vi "Get TDMS File Groups and Channels.vi"(8 "error in":errorcluster, 11 "TDMS ref in":refnum<k34>) -> (0 "error out":errorcluster, 2 "file contents":cluster{string, string[]}[](array[cluster]), 3 "TDMS ref out":refnum<k34>)   [LabVIEW 2020, in "TdmsFileViewer.lvlib"]
uses:
  TdmsFileViewer.lvlib
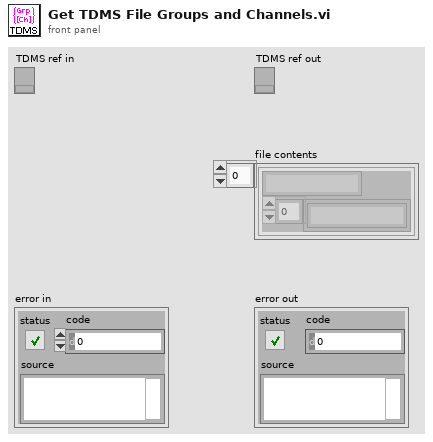
[diagram p1: front panel]
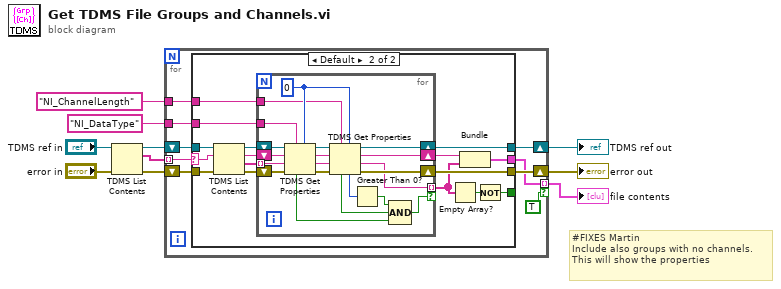
[diagram p0: block diagram]
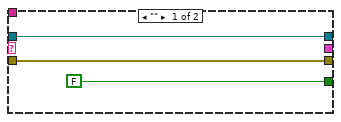
[diagram p2: hidden frame]
diagram:
  # "#FIXES Martin\nInclude also groups with no channels.\nThis will show the properties"
  n1 = TDMS List Contents(4:"error in", 7:"TDMS ref in") -> (0:w9:errorcluster, 2:w3:string[], 3:w2:refnum<k34>)  [unwired: 1 in, 1 out]
  n2 = for {
    tunnel: w3 -> [w17] mode=indexing
    shift-right: [w15] -> w4
    shift-left: w2 -> [w16]
    shift-right: [w18] -> w10
    shift-left: w9 -> [w19]
    tunnel: [w14] -> w5 mode=indexing if=TRUE
    tunnel: "NI_ChannelLength" ("property name") -> [w13]
    tunnel: "NI_DataType" ("property name") -> [w12]
    n3 = case shown="Default" w17 {
      selector: w17 -> [_ w35]
      tunnel: w16 -> [w21 w34]
      tunnel: [w21 w29] -> w15
      tunnel: w19 -> [w22 w38]
      tunnel: [w22 w36] -> w18
      tunnel: [FALSE ("create index file? (T)") w32] -> _
      tunnel: [_ w31] -> w14
      tunnel: w13 -> [_ w25]
      tunnel: w12 -> [_ w24]
      frame "" {
      }
      frame Default {
        n4 = TDMS List Contents(4:w38, 6:w35, 7:w34) -> (0:w37:errorcluster, 1:w27:string[], 2:w28:string, 3:w30:refnum<k34>)
        n5 = for {
          shift-right: [w44] -> w29
          shift-left: w30 -> [w55]
          shift-right: [w56] -> w36
          shift-left: w37 -> [w58]
          tunnel: w27 -> [w53] mode=indexing
          shift-right: [w49] -> w26
          shift-left: w28 -> [w54]
          tunnel: [w48] -> w23 mode=indexing if=w39
          tunnel: w25 -> [w46]
          tunnel: w24 -> [w45]
          w47 = u16 0
          n6 = TDMS Get Properties(5:w47, 7:w45, 8:w58, 9:w53, 10:w54, 11:w55) -> (0:w57:errorcluster, 1:w51:string, 2:w52:string, 3:w50:refnum<k34>, 6:w41:bool)  [unwired: 1 out]
          n7 = TDMS Get Properties(5:w47, 7:w46, 8:w57, 9:w51, 10:w52, 11:w50) -> (0:w56:errorcluster, 1:w48:string, 2:w49:string, 3:w44:refnum<k34>, 4:w43:u16, 6:w42:bool)
          n8 = Greater Than 0?(x=w43) -> (x > 0?=w40:bool)
          n9 = Compound Arithmetic op=AND(w40, w42, w41) -> (w39:bool)
        }
        n10 = Empty Array?(array=w23) -> (empty?=w33:bool)
        n11 = Bundle(w26, w23) -> (w31:cluster{string, string[]})  [unwired: 1 in]
        n12 = Not(x=w33) -> (.not. x?=w32:bool)
      }
    }
  }
  "error out" <- w10
  "file contents" <- w5
  "TDMS ref out" <- w4
